vi "DataStream_PC_Add Name To Map.vi"(7 "Point Size":i32, 9 "Name":string, 11 "Map":map{string, T1}(c390)) -> (3 "Map Out":map{string, T1}(c390))   [LabVIEW 2020]
uses:
  TypeDefs/Cluster_DataStream PC Map Data Set.ctl
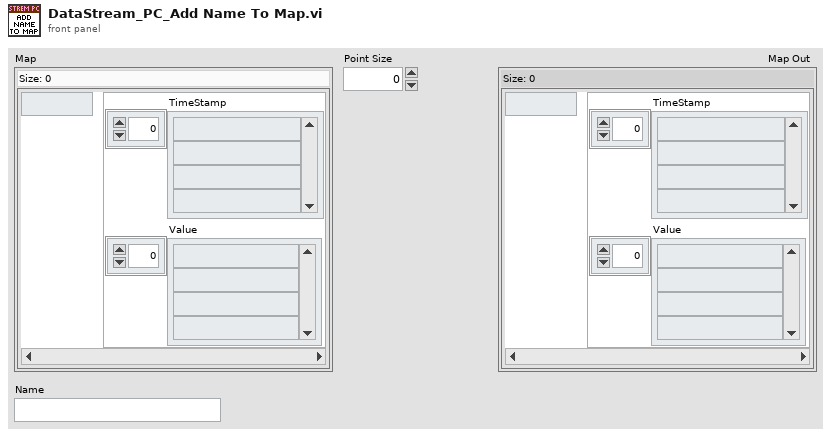
[diagram p1: front panel]
types:
  T1 = typedef "Cluster_DataStream PC Map Data Set.ctl" = cluster{"TimeStamp":dbl[], "Value":dbl[]}
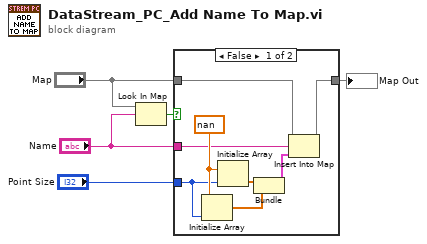
[diagram p0: block diagram]
diagram:
  n1 = Look In Map(map="Map", key="Name") -> (key not found?=w5:bool)  [unwired: 1 in, 1 out]
  n2 = case shown="False" w5 {
    tunnel: "Map" -> [w9 w14]
    tunnel: [w8 w14] -> w3
    tunnel: "Name" -> [w6 _]
    tunnel: "Point Size" -> [w12 _]
    frame False {
      w13 = nan
      n3 = Initialize Array(w13, w12) -> (w10:dbl[])
      n4 = Initialize Array(w13, w12) -> (w11:dbl[])
      n5 = Bundle(w11, w10) -> (w7:cluster{dbl[], dbl[]})  [unwired: 1 in]
      n6 = Insert Into Map(map in=w9, key=w6, value=w7) -> (map out=w8:map{string, T1})  [unwired: 2 out]
    }
    frame True {
    }
  }
  "Map Out" <- w3
